vi "Change Camera.vi"(8 "error in (no error)":errorcluster, 10 "New Camera":string, 11 "HIJ IMAQdx Camera Viewer In":refnum<class "HIJ IMAQdx Camera Viewer.lvclass">) -> (0 "error out":errorcluster, 3 "HIJ IMAQdx Camera Viewer Out":refnum<class "HIJ IMAQdx Camera Viewer.lvclass">)   [LabVIEW 2014, in "HIJ IMAQdx Justage Camera w Timer.lvlib" / "HIJ IMAQdx Camera Viewer.lvclass"]
uses:
  HIJ IMAQdx Camera Viewer.lvclass
  HIJ IMAQdx Camera Viewer.lvclass/HIJ IMAQdx Camera Viewer.ctl
  Applications/HIJ Vision Camera App/HIJ Vision Camera App/HIJ Vision Camera App.lvclass/HIJ Vision Camera App.ctl
  Applications/HIJ Vision Camera App Dialog/HIJ Vision Camera App Dialog Messages/New Camera Selection Msg/New Camera Selection Msg.lvclass/New Camera Selection Msg.ctl
  <vilib>/ActorFramework/Message Enqueuer/Message Enqueuer.lvclass/Message Enqueuer.ctl
  Applications/HIJ Vision Camera App/HIJ Vision Camera App/Read Dialog Enq.vi
  <vilib>/ActorFramework/Message Enqueuer/Enqueue.vi
  <vilib>/ActorFramework/Message Priority Queue/Priority Enqueue.vi
  Applications/HIJ Vision Camera App/HIJ Vision Camera App/HIJ Vision Camera App.lvclass
  <vilib>/ActorFramework/Message Enqueuer/Message Enqueuer.lvclass
  Applications/HIJ Vision Camera App Dialog/HIJ Vision Camera App Dialog Messages/New Camera Selection Msg/New Camera Selection Msg.lvclass
  Shared Code/Viewable Actor/ViewableActor/ViewableActor.lvclass
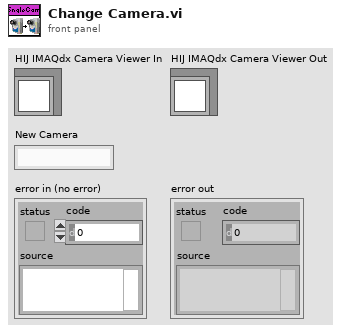
[diagram p1: front panel]
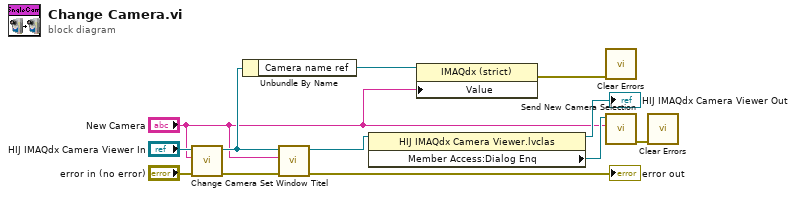
[diagram p0: block diagram]
diagram:
  n1 = call-parent "Change Camera.vi"("error in (no error)"="error in (no error)", "New Camera"="New Camera", "HIJ Vision Camera App In"="HIJ IMAQdx Camera Viewer In") -> ("error out"=w6:errorcluster, "HIJ Vision Camera App Out"=w8:refnum<class "HIJ IMAQdx Camera Viewer.lvclass">)  [unwired: 7 in]
  n2 = Unbundle By Name(w8) -> ("Camera name ref"=w7:refnum<vi>)
  n3 = call "Set Window Titel.vi"("error in (no error)"=w6, "Title"="New Camera", "ViewableActor in"=w8) -> ("error out"=→"error out":errorcluster, "ViewableActor out"=w10:refnum<class "HIJ IMAQdx Camera Viewer.lvclass">)  [unwired: 7 in]
  n4 = property class="HIJ IMAQdx Camera Viewer.lvclas"(reference=w10) -> (reference out=→"HIJ IMAQdx Camera Viewer Out":refnum<class "HIJ IMAQdx Camera Viewer.lvclass">, "Member Access:Dialog Enq"=w3:refnum<class "Message Enqueuer.lvclass">)  [unwired: 1 in, 1 out]
  n5 = property class="IMAQdx (strict)"(reference=w7, "Value"="New Camera") -> (error out=w5:errorcluster)  [unwired: 1 in, 1 out]
  n6 = call <vilib>:"Clear Errors.vi"("error in (no error)"=w5) -> ()  [unwired: 5 in, 2 out]
  n7 = call "Send New Camera Selection.vi"("New Camera Selection"="New Camera", "Message Enqueuer"=w3) -> ("error out"=w1:errorcluster)  [unwired: 8 in, 1 out]
  n8 = call <vilib>:"Clear Errors.vi"("error in (no error)"=w1) -> ()  [unwired: 5 in, 2 out]
